vi "WriteMultipleDigitalOutputs.vi"(8 "error in (no error)":errorcluster, 10 "data":bool[](array[boolean]), 11 "TesteractHAL_DigitalOutput_NIDAQmx In":refnum<class "TesteractHAL_DigitalOutput_NIDAQmx.lvclass">) -> (0 "error out":errorcluster, 3 "TesteractHAL_DigitalOutput_NIDAQmx Out":refnum<class "TesteractHAL_DigitalOutput_NIDAQmx.lvclass">)   [LabVIEW 2017, in "TesteractHAL_DigitalOutput_NIDAQmx.lvlib" / "TesteractHAL_DigitalOutput_NIDAQmx.lvclass"]
doc: "Write multiple lines with a boolean array."
uses:
  TesteractHAL_DigitalOutput_NIDAQmx.lvclass
  TesteractHAL_DigitalOutput_NIDAQmx.lvclass/TesteractHAL_DigitalOutput_NIDAQmx.ctl
  <vilib>/DAQmx/write.llb/DAQmx Write (Digital 1D Bool 1Chan 1Samp).vi
  <vilib>/DAQmx/create/channels.llb/DAQmx Create Channel (DO-Digital Output).vi
  <vilib>/DAQmx/miscellaneous.llb/DAQmx Fill In Error Info.vi
  <resource>/objmgr/daqmx.rc
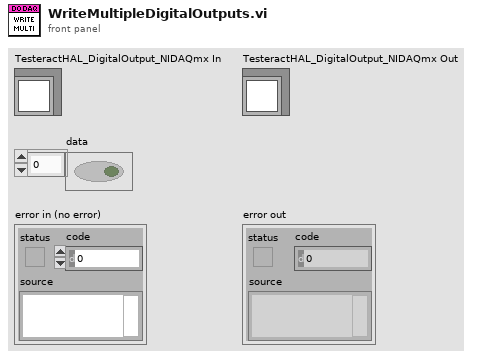
[diagram p1: front panel]
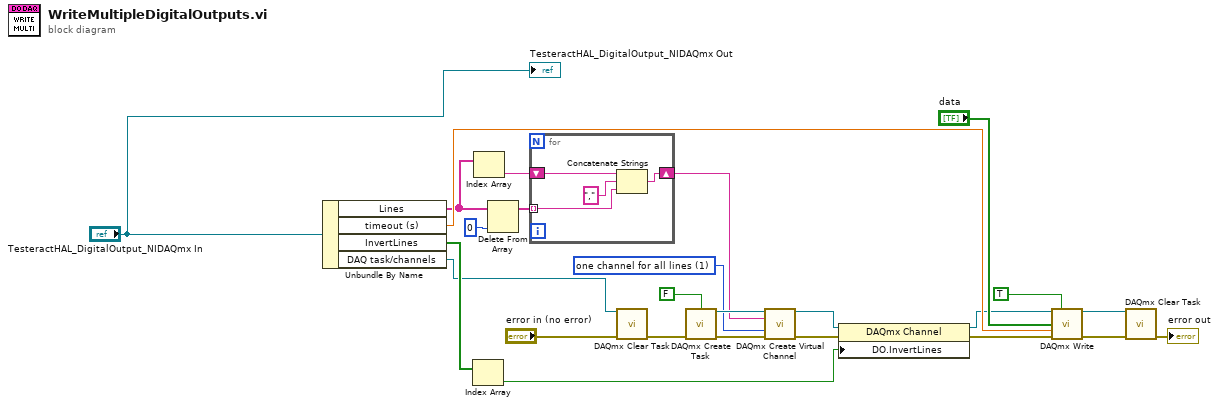
[diagram p0: block diagram]
diagram:
  w10 = 1 items=["one channel for each line", "one channel for all lines"] ("line grouping")
  n1 = Unbundle By Name("TesteractHAL_DigitalOutput_NIDAQmx In") -> ("Lines"=w9:string[], "timeout (s)"=w21:dbl, "InvertLines"=w8:bool[], "DAQ task/channels"=w3:refnum<k21>)
  n2 = Index Array(array=w8) -> (element=w11:bool)  [unwired: 1 in]
  n3 = Index Array(array=w9) -> (element=w14:string)  [unwired: 1 in]
  n4 = Delete From Array(array=w9, index=0) -> (array with subset deleted=w13:string[])  [unwired: 1 in, 1 out]
  n5 = for {
    shift-right: [w28] -> w12
    shift-left: w14 -> [w27]
    tunnel: w13 -> [w26] mode=indexing
    n6 = Concatenate Strings(w27, ",", w26) -> (w28:string)
  }
  n7 = call <vilib>:"DAQmx Clear Task.vi"("task in"=w3, "error in"="error in (no error)") -> ("error out"=w1:errorcluster)  [unwired: 13 in]
  n8 = call <vilib>:"DAQmx Create Task.vi"("auto cleanup"=FALSE, "error in"=w1) -> ("task out"=w19:refnum<k21>, "error out"=w20:errorcluster)  [unwired: 12 in]
  n9 = call-poly <vilib>:"DAQmx Create Virtual Channel.vi"("task in"=w19, "lines"=w12, "line grouping"=w10, "error in"=w20) -> ("task out"=w16:refnum<k21>, "error out"=w17:errorcluster)  [unwired: 10 in]
  n10 = property class="DAQmx Channel"(reference=w16, error in=w17, "DO.InvertLines"=w11) -> (reference out=w6:refnum<k21>, error out=w7:errorcluster)
  n11 = call-poly <vilib>:"DAQmx Write.vi"("task/channels in"=w6, "auto start"=TRUE, "data"="data", "timeout"=w21, "error in"=w7) -> ("task out"=w4:refnum<k21>, "error out"=w23:errorcluster)  [unwired: 8 in, 1 out]
  n12 = call <vilib>:"DAQmx Clear Task.vi"("task in"=w4, "error in"=w23) -> ("error out"=→"error out":errorcluster)  [unwired: 13 in]
  "TesteractHAL_DigitalOutput_NIDAQmx Out" <- "TesteractHAL_DigitalOutput_NIDAQmx In"
